vi "TestNoLibrary.vi"   [LabVIEW 2018]
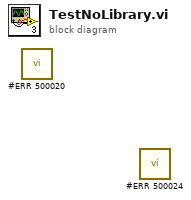
[diagram p0: block diagram]
diagram:
  n1 = call "#ERR 500020"() -> ()  [unwired: 11 in, 1 out]
  n2 = call "#ERR 500024"() -> ()  [unwired: 11 in, 1 out]
